vi "CameraAttributeTest.vi"() -> ()   [LabVIEW 2024]
uses:
  <vilib>/userDefined/High Color/IMAQdx.ctl
  <vilib>/vision/driver/NI_Vision_Acquisition_Software.lvlib
  <resource>/objmgr/imaqdx.rc
panel:
  out "Array":errorcluster[](array[cluster])
  out "Numeric":i32
  in  "Session In":T1
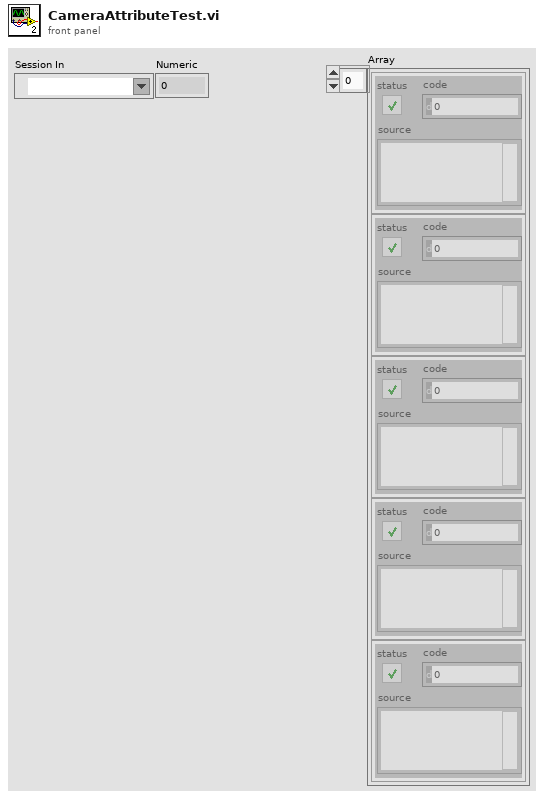
[diagram p1: front panel]
types:
  T1 = typedef "IMAQdx.ctl" = refnum<k21>
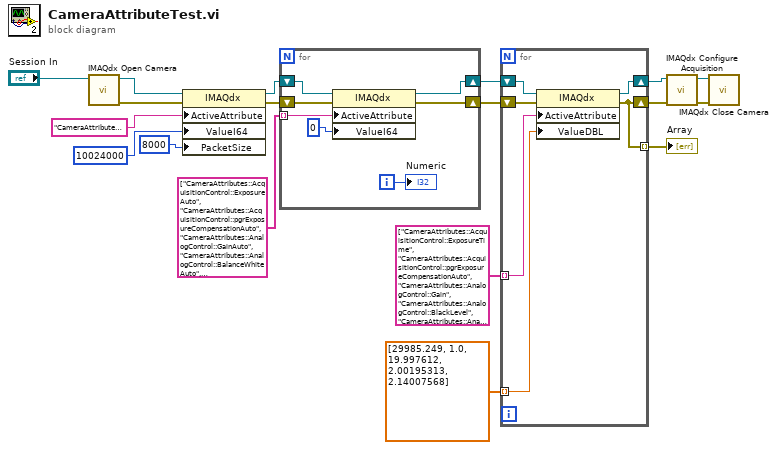
[diagram p0: block diagram]
diagram:
  n1 = call <vilib>:"IMAQdx Open Camera.vi"("Session In"="Session In") -> ("error out"=w11:errorcluster, "Session Out"=w12:T1)  [unwired: 9 in]
  n2 = property class="IMAQdx"(reference=w12, error in=w11, "ActiveAttribute"="CameraAttributes::DeviceControl::DeviceLinkThroughputLimit", "ValueI64"=i64 10024000, "PacketSize"=u32 8000) -> (reference out=w8:T1, error out=w9:errorcluster)
  n3 = for {
    tunnel: string[] ["CameraAttributes::AcquisitionControl::ExposureAuto", "CameraAttributes::AcquisitionControl::pgrExposureCompensationAuto", "CameraAttributes::AnalogControl::GainAuto", "CameraAttributes::AnalogControl::BalanceWhiteAuto", "CameraAttributes::AnalogControl::BalanceRatioSelector"] -> [w24] mode=indexing
    shift-right: [w20] -> w5
    shift-left: w8 -> [w21]
    shift-right: [w19] -> w4
    shift-left: w9 -> [w22]
    i -> [w23]
    n4 = property class="IMAQdx"(reference=w21, error in=w22, "ActiveAttribute"=w24, "ValueI64"=i64 0) -> (reference out=w20:T1, error out=w19:errorcluster)
    "Numeric" <- w23
  }
  n5 = for {
    shift-right: [w29] -> w3
    shift-left: w5 -> [w31]
    shift-right: [w26] -> w2
    shift-left: w4 -> [w30]
    tunnel: string[] ["CameraAttributes::AcquisitionControl::ExposureTime", "CameraAttributes::AcquisitionControl::pgrExposureCompensationAuto", "CameraAttributes::AnalogControl::Gain", "CameraAttributes::AnalogControl::BlackLevel", "CameraAttributes::AnalogControl::BalanceRatio"] -> [w28] mode=indexing
    tunnel: dbl[] [29985.249, 1.0, 19.997612, 2.00195313, 2.14007568] -> [w27] mode=indexing
    tunnel: [w26] -> w1 mode=indexing
    n6 = property class="IMAQdx"(reference=w31, error in=w30, "ActiveAttribute"=w28, "ValueDBL"=w27) -> (reference out=w29:T1, error out=w26:errorcluster)
  }
  "Array" <- w1
  n7 = call <vilib>:"IMAQdx Configure Acquisition.vi"("error in"=w2, "Session In"=w3) -> ("error out"=w16:errorcluster, "Session Out"=w17:T1)  [unwired: 8 in]
  n8 = call <vilib>:"IMAQdx Close Camera.vi"("error in"=w16, "Session In"=w17) -> ()  [unwired: 9 in, 1 out]
